vi "BuildBase64StringFromImage.vi"(8 "error in":errorcluster, 11 "path":path) -> (0 "error out":errorcluster, 3 "concatenated string":string)   [LabVIEW 2018, in "feGEM DataPacker.lvlib"]
uses:
  feGEM DataPacker.lvlib
panel:
  out "Image Base64 String":string
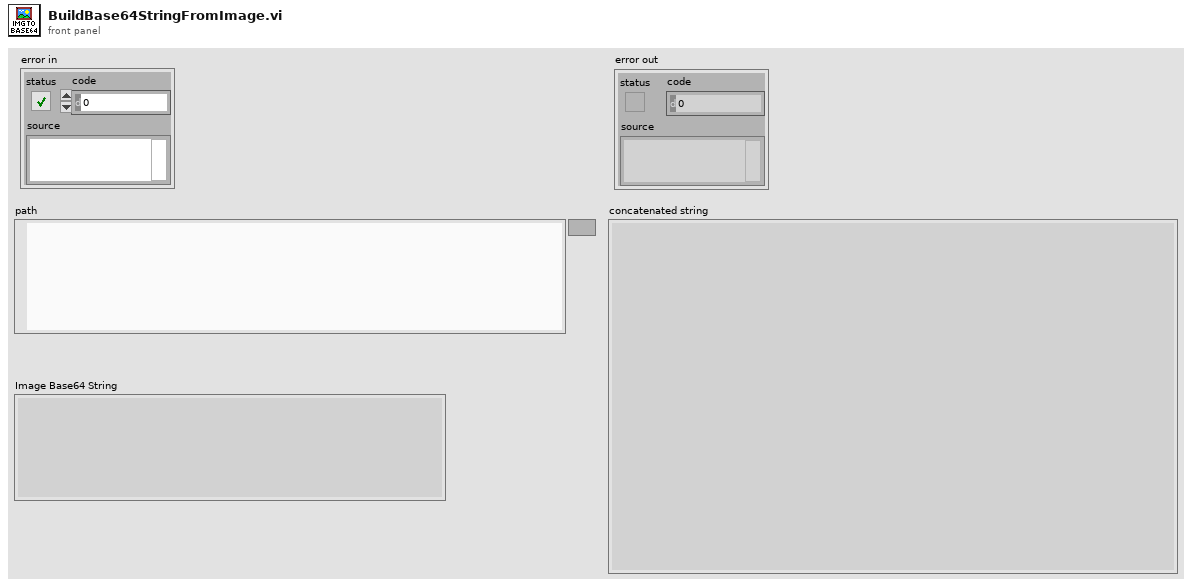
[diagram p1: front panel]
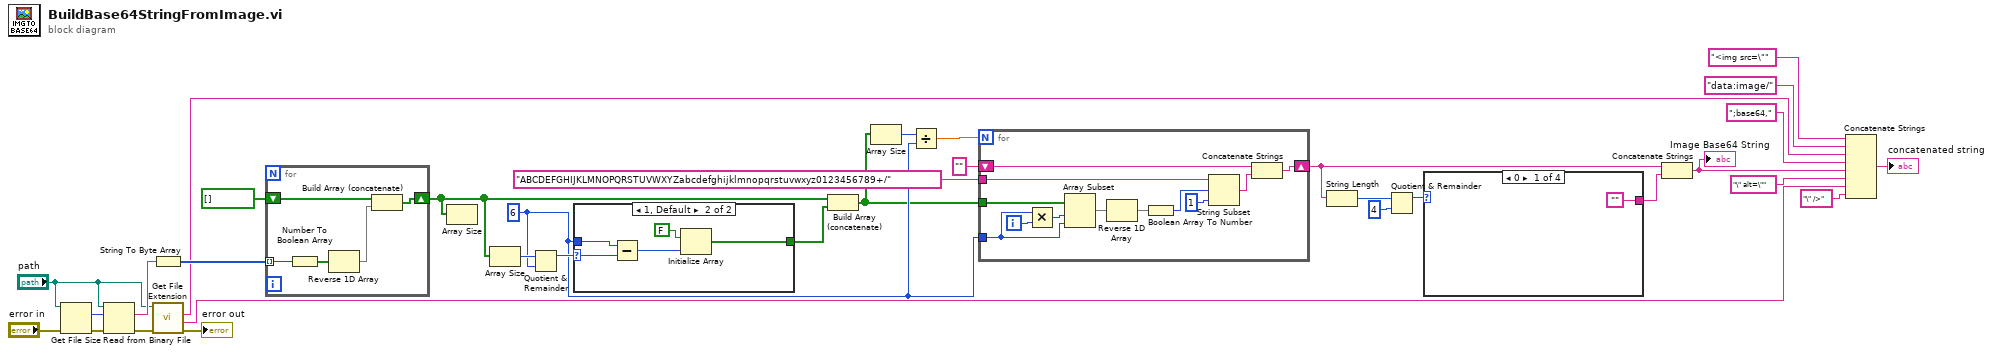
[diagram p0: block diagram]
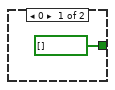
[diagram p2: hidden frame]
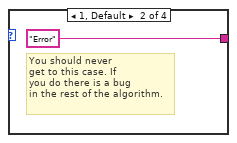
[diagram p3: hidden frame]
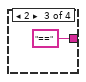
[diagram p4: hidden frame]
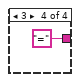
[diagram p5: hidden frame]
diagram:
  w20 = 6 ("y")
  n1 = Get File Size(file="path", error in="error in") -> (size (in bytes)=w9:i64, 0:w8:errorcluster)  [unwired: 1 out]
  n2 = Read from Binary File(8:w8, 10:w9, 11:"path") -> (0:w6:errorcluster, 2:w11:string)  [unwired: 3 in, 2 out]
  n3 = String To Byte Array(string=w11) -> (unsigned byte array=w33:u8[])
  n4 = call <vilib>:"Get File Extension.vi"("error in (no error)"=w6, "file"="path") -> ("error out"=→"error out":errorcluster, "filename without extension"=w1:string, "lowercase file extension"=w12:string)  [unwired: 5 in, 2 out]
  n5 = for {
    tunnel: w33 -> [w38] mode=indexing
    shift-right: [w35] -> w17
    shift-left: bool[] [] -> [w37]
    n6 = Number To Boolean Array(number=w38) -> (Boolean array=w36:bool[])
    n7 = Reverse 1D Array(array=w36) -> (reversed array=w34:bool[])
    n8 = Build Array (concatenate)(w37, w34) -> (w35:bool[])
  }
  n9 = Array Size(array=w17) -> ()  [unwired: 1 out]
  n10 = Array Size(array=w17) -> (size(s)=w23:i32)
  n11 = Quotient & Remainder(x=w23, y=w20) -> (x-y*floor(x/y)=w22:i32)  [unwired: 1 out]
  n12 = case shown="1, Default" w22 {
    selector: w22 -> [_ w43]
    tunnel: [bool[] [] w40] -> w21
    tunnel: w20 -> [_ w42]
    frame 0 {
    }
    frame 1, Default {
      n13 = Subtract(x=w42, y=w43) -> (x-y=w44:i32)
      n14 = Initialize Array(FALSE, w44) -> (w40:bool[])
    }
  }
  n15 = Build Array (concatenate)(w17, w21) -> (w19:bool[])
  n16 = Array Size(array=w19) -> (size(s)=w18:i32)
  n17 = Divide(x=w18, y=w20) -> (x/y=w24:dbl)
  n18 = for {
    N: w24 -> [_]
    tunnel: w19 -> [w55]
    tunnel: w20 -> [w53]
    tunnel: "ABCDEFGHIJKLMNOPQRSTUVWXYZabcdefghijklmnopqrstuvwxyz0123456789+/" -> [w52]
    shift-right: [w50] -> w25
    shift-left: "" -> [w49]
    i -> [w56]
    n19 = Multiply(x=w53, y=w56) -> (x*y=w54:i32)
    n20 = Array Subset(array=w55, index=w54, length=w53) -> (w45:bool[])
    n21 = Reverse 1D Array(array=w45) -> (reversed array=w46:bool[])
    n22 = Boolean Array To Number(Boolean array=w46) -> (number=w47:u32)
    n23 = String Subset(string=w52, offset (0)=w47, length (rest)=1 ("length (rest)")) -> (substring=w48:string)
    n24 = Concatenate Strings(w49, w48) -> (w50:string)
  }
  n25 = String Length(string=w25) -> (length=w29:i32)
  n26 = Quotient & Remainder(x=w29, y=4) -> (x-y*floor(x/y)=w27:i32)  [unwired: 1 out]
  n27 = case shown="0" w27 {
    tunnel: ["" "Error" "==" "="] -> w26
    frame 0 {
    }
    frame 1, Default {
      # "You should never\nget to this case. If\nyou do there is a bug\nin the rest of the algorithm."
    }
    frame 2 {
    }
    frame 3 {
    }
  }
  n28 = Concatenate Strings(w25, w26) -> (w16:string)
  "Image Base64 String" <- w16
  n29 = Concatenate Strings("<img src=\"", "data:image/", w12, ";base64,", w16, "\" alt=\"" ("string"), w1, "\" />" ("string")) -> (→"concatenated string":string)
